vi "Close File.vi"(8 "error in (no error)":errorcluster, 11 "Data In":T1) -> (0 "error out":errorcluster, 3 "Data Out":T1)   [LabVIEW 2010, in "TDMS Custom Device.lvlib"]
uses:
  TDMS Custom Device.lvlib
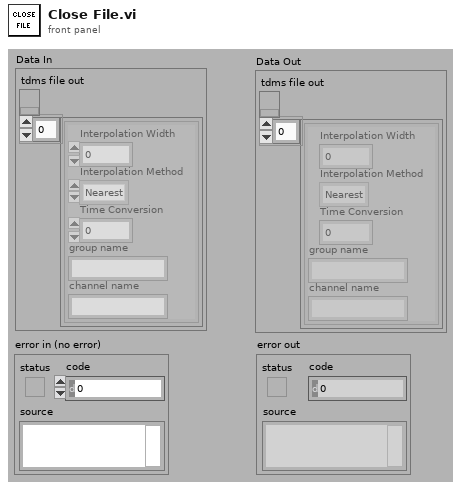
[diagram p1: front panel]
types:
  T1 = cluster{"tdms file out":refnum<k34>, cluster{"Interpolation Width":i32, "Interpolation Method":enum16{"Nearest", "Linear", "Spline", "Cubic Hermite", "Lagrange", "Polynomial"}, "Time Conversion":dbl, "group name":string, "channel name":string}[]}
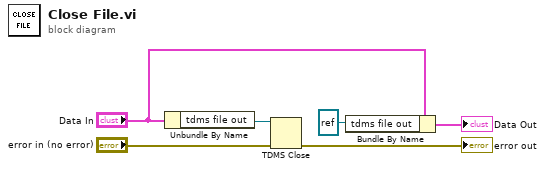
[diagram p0: block diagram]
diagram:
  n1 = Unbundle By Name("Data In") -> ("tdms file out"=w6:refnum<k34>)
  n2 = TDMS Close(8:"error in (no error)", 11:w6) -> (0:→"error out":errorcluster)  [unwired: 1 out]
  n3 = Bundle By Name(cluster="Data In", "tdms file out"=refnum<k34> refnum) -> (→"Data Out":T1)
